vi "Image Acquiring Module.vi"(7 "Scan Status in":enum16{"Start", "Continue Scan", "Finish Scan"}(ring), 8 "Error in":errorcluster, 10 "Channel":u32(ring)=1 items=["A"=1, "B"=2, "A + B"=3, "C"=4, "A + C"=5, "A + B"=6, "D"=8, "A + D"=9, "B + D"=10, "C + D"=12, "A + B + C + D"=15], 11 "Quit?":bool=TRUE) -> (0 "Error Out":errorcluster)   [LabVIEW 2018]
uses:
  Controls/QueueNames.ctl
  Controls/MessagePacket.ctl
  Controls/Queue Manager Actions.ctl
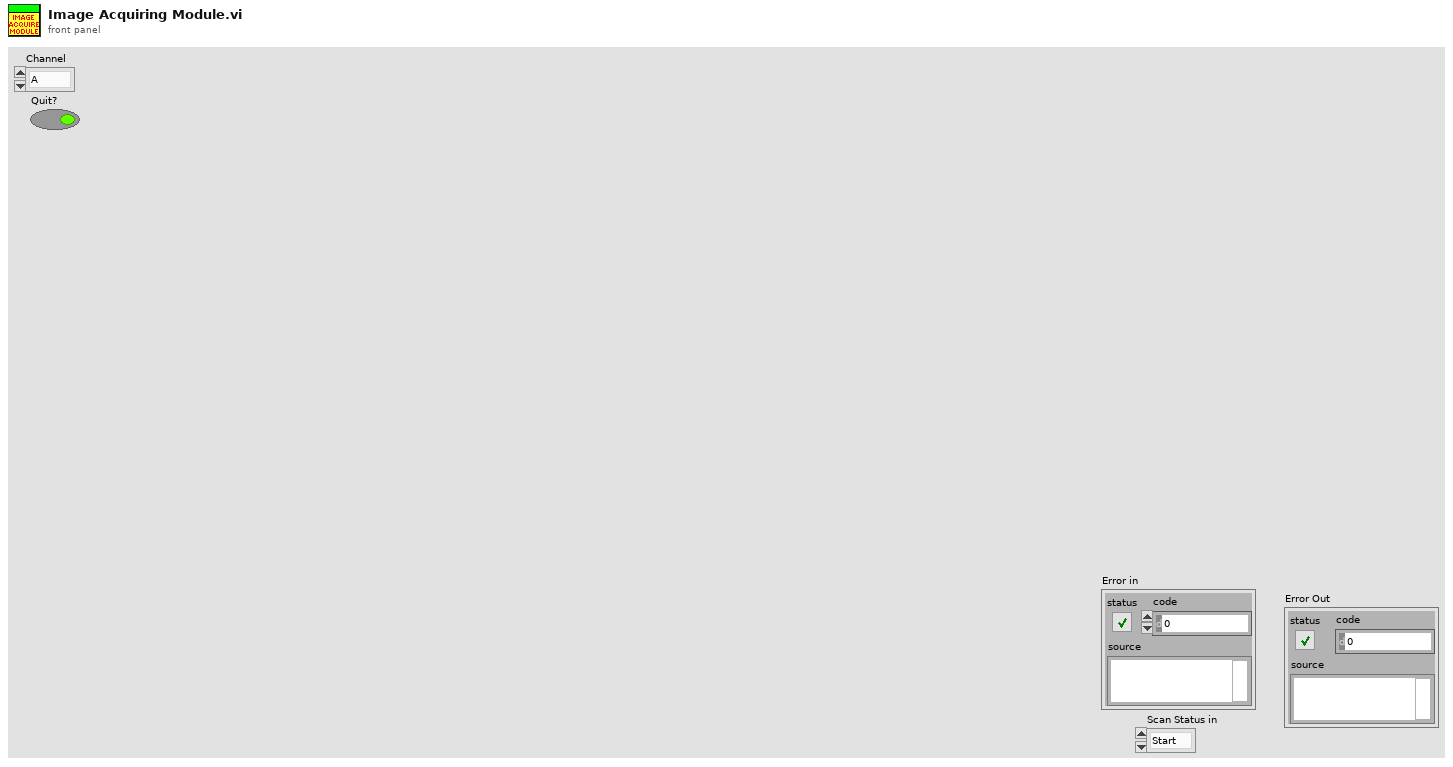
[diagram p1: front panel]
types:
  T1 = typedef "Queue Manager Actions.ctl" = enum16{"Init", "Enqueue", "Enqueue All", "Preview Queue", "Dequeue", "Get Status", "Flush Queue", "Flush All Queues", "Release All Queues", "Release Queue", "Enqueue at Opposite End"}
  T2 = typedef "MessagePacket.ctl" = cluster{"Message":string, "Parameter":variant}
  T3 = typedef "QueueNames.ctl" = enum16{"Main GUI", "Main Scan Processor", "Main Processing", "Main Saving", "Main Display", "Main Table Stage GUI", "Main Table Stage Proc.", "Scan Engine", "Vibratome GUI", "Vibratome Processor", "Slice Engine"}
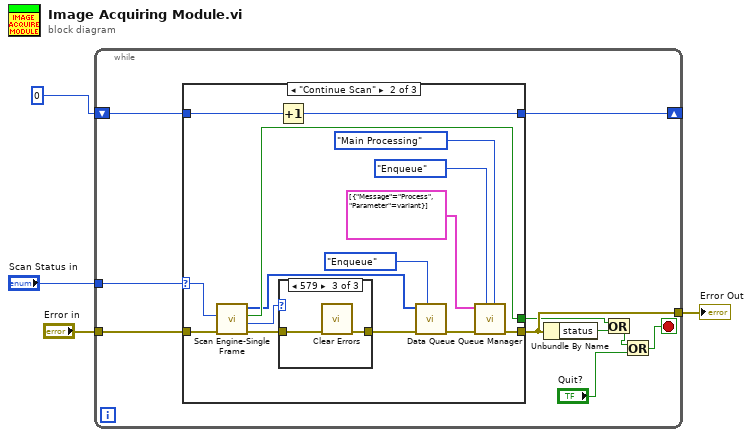
[diagram p0: block diagram]
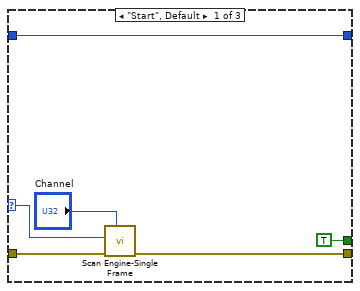
[diagram p2: hidden frame]
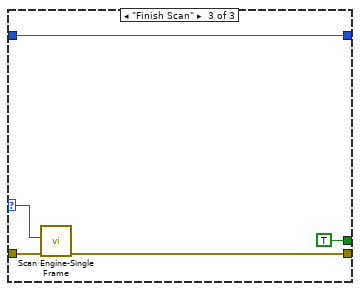
[diagram p5: hidden frame]
diagram:
  n1 = while {
    tunnel: "Error in" -> [w12]
    tunnel: "Scan Status in" -> [w14]
    tunnel: [w11] -> w2
    shift-right: [w13] -> _
    shift-left: u32 0 ("t") -> [w8]
    stop <- w6 stop-if-true
    n2 = case shown="\"Continue Scan\"" w14 {
      selector: w14 -> [w19 w34 w44]
      tunnel: w12 -> [w20 w35 w43]
      tunnel: [w17 w32 w40] -> w11
      tunnel: [TRUE w33 TRUE ("task done?")] -> w9
      tunnel: w8 -> [w15 w26 w41]
      tunnel: [w15 w25 w41] -> w13
      frame "Start", Default {
        n3 = call "Scan Engine-Single Frame.vi"("Channel"="Channel", "Error in"=w20, "Scan Status"=w19) -> ("Error Out"=w17:errorcluster)  [unwired: 5 in, 3 out]
      }
      frame "Continue Scan" {
        n4 = call "Scan Engine-Single Frame.vi"("Error in"=w35, "Scan Status"=w34) -> ("Error Out"=w24:errorcluster, "Return Code"=w22:u32, "task done?"=w33:bool, "data out"=w21:u16[])  [unwired: 6 in]
        n5 = Increment(x=w26) -> (x+1=w25:u32)
        n6 = case shown="579" w22 {
          tunnel: w24 -> [w36 w37 w39]
          tunnel: [w36 w37 w38] -> w23
          frame 0 {
          }
          frame 1, Default {
          }
          frame 579 {
            n7 = call <vilib>:"Clear Errors.vi"("error in (no error)"=w39) -> ("error out"=w38:errorcluster)  [unwired: 5 in, 1 out]
          }
        }
        n8 = call "Data Queue.vi"("Action"=Queue_Manager_Actions."Enqueue", "error in (no error)"=w23, "data in"=w21) -> ("error out"=w27:errorcluster)  [unwired: 6 in, 2 out]
        n9 = call "Queue Manager.vi"("Queue Name"=QueueNames."Main Processing", "Action"=Queue_Manager_Actions."Enqueue", "Error In"=w27, "Message Packet Array"=T2[] [{"Message"="Process", "Parameter"=variant}]) -> ("Error Out"=w32:errorcluster)  [unwired: 3 in, 4 out]
      }
      frame "Finish Scan" {
        n10 = call "Scan Engine-Single Frame.vi"("Error in"=w43, "Scan Status"=w44) -> ("Error Out"=w40:errorcluster)  [unwired: 6 in, 3 out]
      }
    }
    n11 = Unbundle By Name(w11) -> ("status"=w10:bool)
    n12 = Or(x=w9, y=w10) -> (x .or. y?=w7:bool)
    n13 = Or(x=w7, y="Quit?") -> (x .or. y?=w6:bool)
  }
  "Error Out" <- w2
